vi "Convert Analog to Channel Settings.vi"(10 "channel default values":dbl[](array[numeric]), 11 "channel names":string[](array[string])) -> (3 "channel settings":T1[](array[typedef]))   [LabVIEW 2017, in "Scan Engine Scripting.lvlib"]
uses:
  Scan Engine Scripting.lvlib
  Modules/Mode Classes/Controls/analog channel settings.ctl
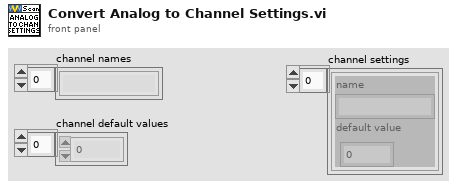
[diagram p1: front panel]
types:
  T1 = typedef "Scan Engine Scripting.lvlib/analog channel settings.ctl" = cluster{"name":string, "default value":dbl}
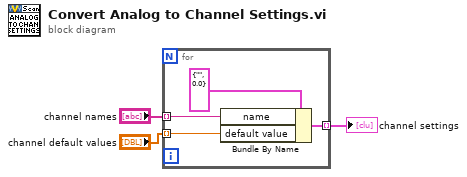
[diagram p0: block diagram]
diagram:
  n1 = for {
    tunnel: "channel names" -> [w6] mode=indexing
    tunnel: "channel default values" -> [w4] mode=indexing
    tunnel: [w5] -> w3 mode=indexing
    n2 = Bundle By Name(cluster=T1 {"name"="", "default value"=0.0} ("channel settings"), "name"=w6, "default value"=w4) -> (w5:T1)
  }
  "channel settings" <- w3
